vi "Append Image File.vi"(0 "PDF Report IN":refnum<class "PDF Report Class.lvclass">, 1 "Scale (%)":sgl=100.0, 3 "Border":T3={"Show?"=FALSE, "Thickness (point)"=0.5, "Color"=0}, 5 "Image path":path, 11 "error in (no error)":errorcluster, 12 "Caption":string, 14 "Position and indentation":T1={"Alignment"=enum."Center", "X "=0.0, "Y"=0.0, "Indentation"=0.0}) -> (4 "PDF Report OUT":refnum<class "PDF Report Class.lvclass">, 6 "Image path duplicate":path, 8 "Size (points)":cluster{"TotalHeight":sgl, "TotalWidth":sgl}, 15 "error out":errorcluster)   [LabVIEW 2019]
doc: "The <B>VI</B> appends, to the PDF report, the image from a file. \n\nValid formats: GIF, JPEG, PNG and BMP.\n\n<B>FRANÇAIS</B>\nLe <B>VI</B> ajoute, au rapport PDF, l'image provenant d'un fichier.\n\nFormats valides : GIF, JPEG, PNG et BMP.\n\nVersion 1.0\nDeveloped by Jean-Marc Simard\nCopyright © 2010, Exaprom Inc.\nAll rights reserved.\nLicense: BSD\n\nWith iTextSharp 4.1.6 (http://itextsharp.sourceforge.net)\nunder Mozilla Public License Version 1.1\n(http://www.mozilla.org/MPL/MPL-1.1.html)"
uses:
  <userlib>/Exaprom PDF/LV Class/PDF Report Class/PDF Report Class.lvclass
  <userlib>/Exaprom PDF/Controls/Image Controls/Image border.ctl
  <userlib>/Exaprom PDF/Controls/Image Controls/Image alignment and position.ctl
  <userlib>/Exaprom PDF/Controls/Image Controls/Image aligment.ctl
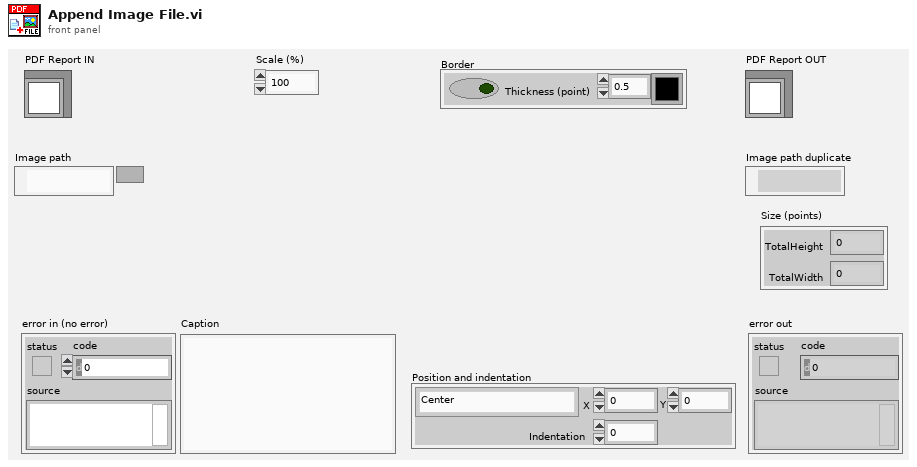
[diagram p1: front panel]
types:
  T1 = typedef "Image alignment and position.ctl" = cluster{"Alignment":T2, "X ":sgl, "Y":sgl, "Indentation":sgl}
  T2 = typedef "Image aligment.ctl" = enum16{"Absolute (X,Y)", "Left", "Center", "Right", "Left (textwrap)", "Right (textwrap)"}
  T3 = typedef "Image border.ctl" = cluster{"Show?":bool, "Thickness (point)":sgl, "Color":u32}
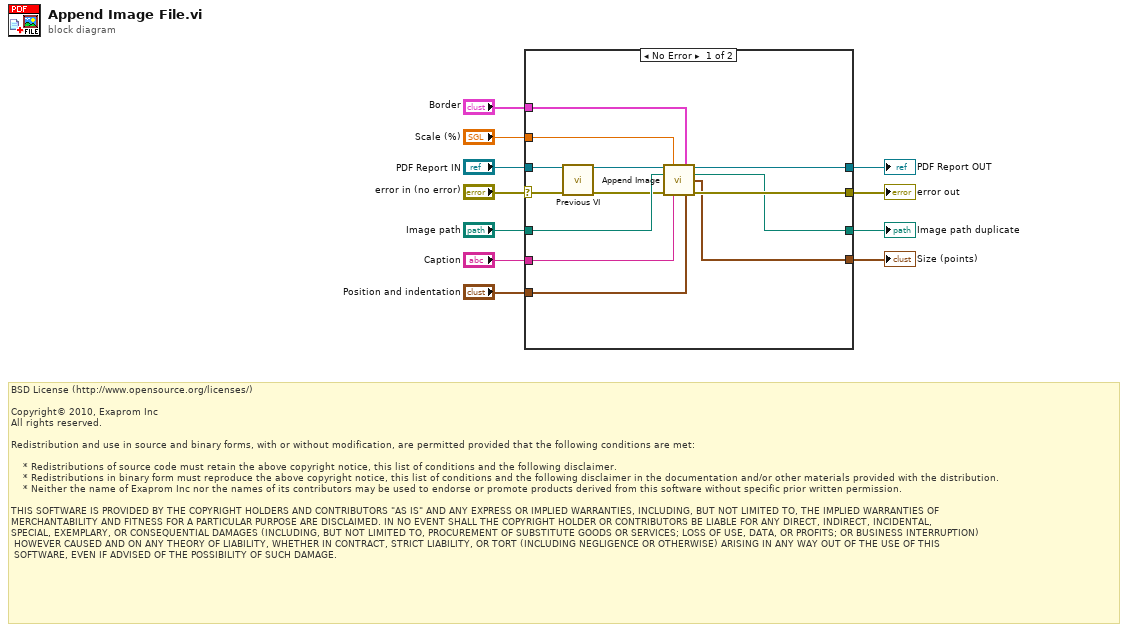
[diagram p0: block diagram]
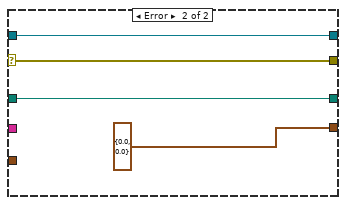
[diagram p2: hidden frame]
diagram:
  # "BSD License (http://www.opensource.org/licenses/)\n\nCopyright© 2010, Exaprom Inc\nAll rights reserved.\n\nRedistribution and use in source and binary forms, with or without modification, are permitted provided that the following conditions are met:\n\n    * Redistributions of source code must retain the above copyright notice, this list of conditions and the following disclaimer.\n    * Redistributions in binary form must reproduce the above copyright notice, this list of conditions and the following disclaimer in the documentation and/or other materials provided with the distribution.\n    * Neither the name of Exaprom Inc nor the names of its contributors may be used to endorse or promote products derived from this software without specific prior written permission.\n\nTHIS SOFTWARE IS PROVIDED BY THE COPYRIGHT HOLDERS AND CONTRIBUTORS \"AS IS\" AND ANY EXPRESS OR IMPLIED WARRANTIES, INCLUDING, BUT NOT LIMITED TO, THE IMPLIED WARRANTIES OF \nMERCHANTABILITY AND FITNESS FOR A PARTICULAR PURPOSE ARE DISCLAIMED. IN NO EVENT SHALL THE COPYRIGHT HOLDER OR CONTRIBUTORS BE LIABLE FOR ANY DIRECT, INDIRECT, INCIDENTAL,\nSPECIAL, EXEMPLARY, OR CONSEQUENTIAL DAMAGES (INCLUDING, BUT NOT LIMITED TO, PROCUREMENT OF SUBSTITUTE GOODS OR SERVICES; LOSS OF USE, DATA, OR PROFITS; OR BUSINESS INTERRUPTION)\n HOWEVER CAUSED AND ON ANY THEORY OF LIABILITY, WHETHER IN CONTRACT, STRICT LIABILITY, OR TORT (INCLUDING NEGLIGENCE OR OTHERWISE) ARISING IN ANY WAY OUT OF THE USE OF THIS\n SOFTWARE, EVEN IF ADVISED OF THE POSSIBILITY OF SUCH DAMAGE."
  n1 = case shown="No Error" "error in (no error)" {
    selector: "error in (no error)" -> [w12 w28]
    tunnel: [w23 w27] -> w6
    tunnel: [w22 w28] -> w11
    tunnel: "PDF Report IN" -> [w24 w27]
    tunnel: "Image path" -> [w19 w26]
    tunnel: [w18 w26] -> w8
    tunnel: "Caption" -> [w16 _]
    tunnel: "Border" -> [w21 _]
    tunnel: "Position and indentation" -> [w15 _]
    tunnel: "Scale (%)" -> [w20 _]
    tunnel: [w17 cluster{"TotalHeight":sgl, "TotalWidth":sgl} {"TotalHeight"=0.0, "TotalWidth"=0.0}] -> w1
    frame No Error {
      n2 = call <userlib>:"Previous VI.vi"("PDF Report IN"=w24, "error in (no error)"=w12) -> ("PDF Report OUT"=w14:refnum<class "PDF Report Class.lvclass">, "error out"=w13:errorcluster)  [unwired: 12 out]
      n3 = call <userlib>:"Append Image.vi"("PDF Report IN"=w14, "Scale (%)"=w20, "Border"=w21, "Image path"=w19, "error in (no error)"=w13, "Caption"=w16, "Position and indentation"=w15) -> ("PDF Report OUT"=w23:refnum<class "PDF Report Class.lvclass">, "Image path duplicate"=w18:path, "Size (points)"=w17:cluster{"TotalHeight":sgl, "TotalWidth":sgl}, "error out"=w22:errorcluster)  [unwired: 1 in, 4 out]
    }
    frame Error {
    }
  }
  "error out" <- w11
  "PDF Report OUT" <- w6
  "Image path duplicate" <- w8
  "Size (points)" <- w1
